vi "Width test.vi"(7 "error in":errorcluster) -> (27 "error out":errorcluster)   [LabVIEW 2014]
panel:
  in  "File Path":path=path "D:/leizhihong/胶水图片/透明胶水检测/IMG0003.bmp"
  in  "Settings":T1={"Contrast"=60, "Filter width"=5, "Steepness"=13, "Subsampling Ratio"=25, "Show Search Area"=TRUE, "Show Search Lines"=TRUE, "Show Edges Found"=TRUE, "Show Result"=TRUE}
  out "Distance":sgl
  in  "确定":bool
  in  "ROI":bool
  in  "停止":bool
  out "Image Out":T2(plugin-control)
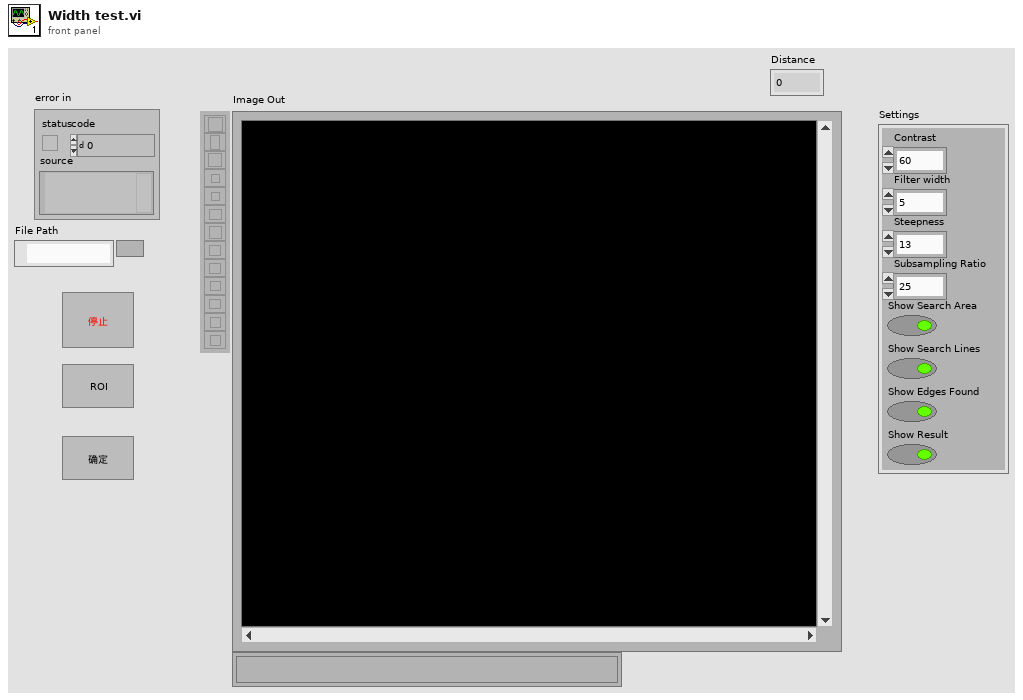
[diagram p1: front panel]
types:
  T1 = cluster{"Contrast":i32, "Filter width":i32, "Steepness":i32, "Subsampling Ratio":u32, "Show Search Area":bool, "Show Search Lines":bool, "Show Edges Found":bool, "Show Result":bool}
  T2 = typedef "IMAQ Image.ctl" = refnum<image>
  T3 = typedef "Image Type" = u32
  T4 = cluster{"Global Rectangle":i32[], "Contours":cluster{"Contour Type":u32, "ROI Type":u32, "Points":i32[]}[]}
  T5 = cluster{"Global Rectangle":i32[], "Contours":cluster{"ID":enum32{"External", "Internal"}, "Type":u32, "Coordinates":i32[]}[]}
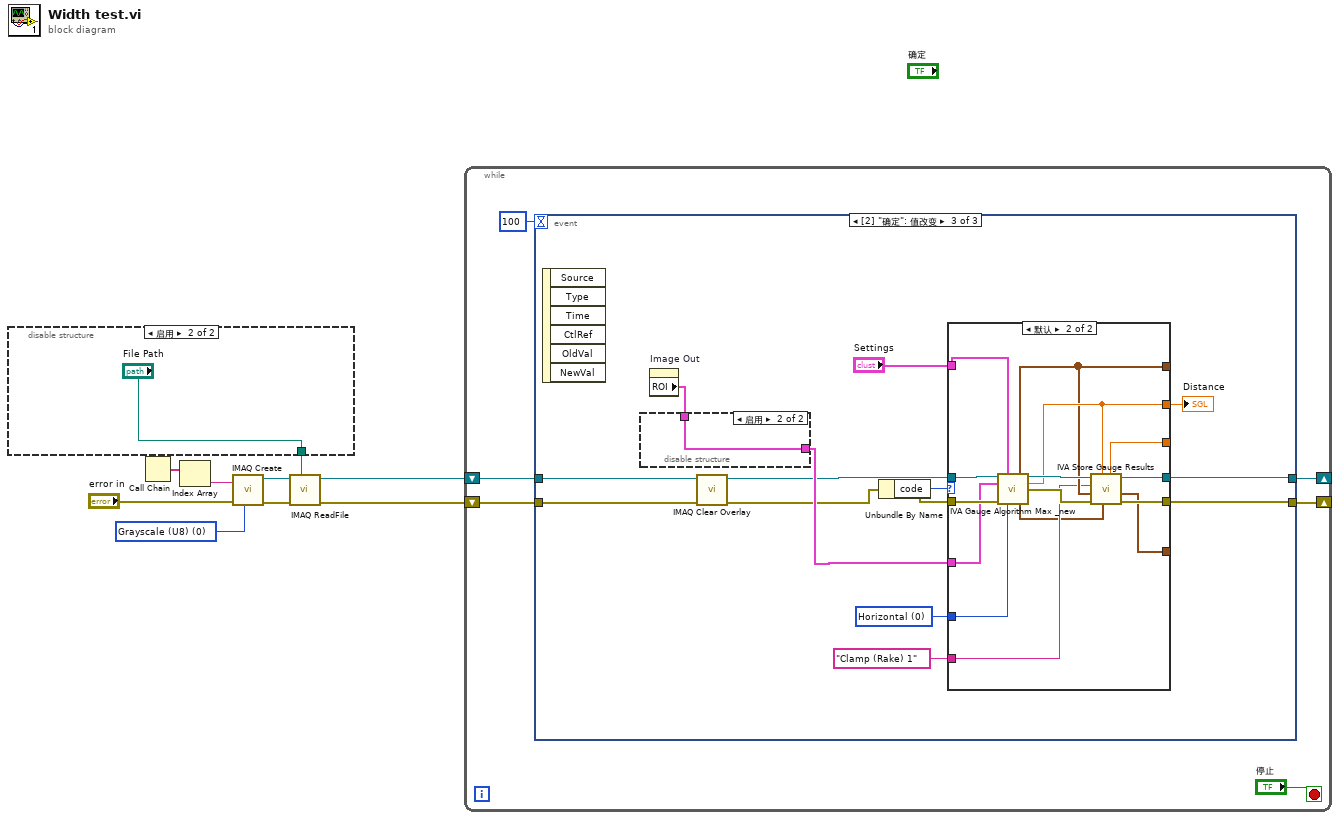
[diagram p0: block diagram]
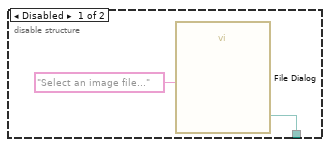
[diagram p2: hidden frame]
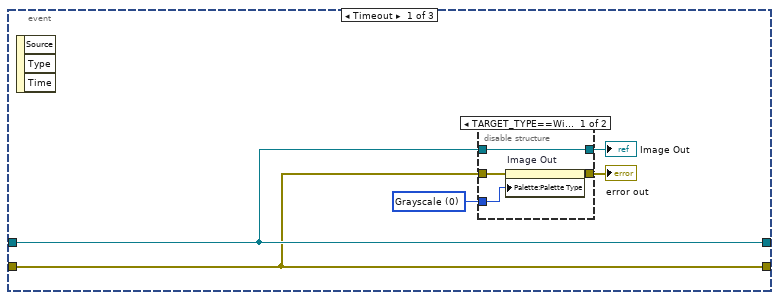
[diagram p3: hidden frame]
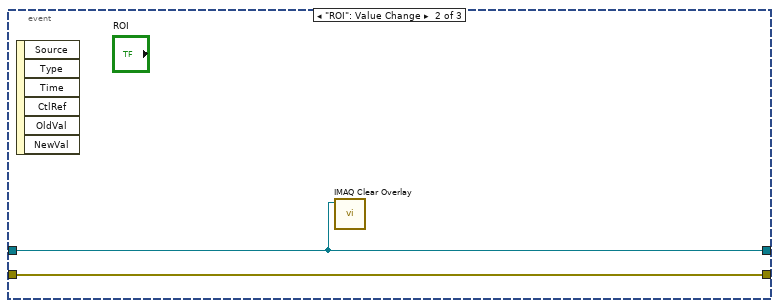
[diagram p5: hidden frame]
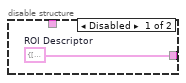
[diagram p6: hidden frame]
diagram:
  w2 = T3 0 items=["Grayscale (U8)", "Grayscale (I16)", "Grayscale (SGL)", "Complex (CSG)", "RGB (U32)", "HSL (U32)", "RGB (U64)", "Grayscale (U16)"] ("Image Type")
  n1 = disable-structure shown="启用" {
    disable-tunnel: [w10 "File Path"] -> w3
    frame Disabled {
      n2 = call "File Dialog"("prompt"="Select an image file...") -> ("selected path"=w10:path)  [unwired: 6 in, 8 out]
    }
    frame Enabled {
    }
  }
  n3 = Call Chain() -> (call chain=w5:string[])
  n4 = Index Array(array=w5) -> (element=w4:string)  [unwired: 1 in]
  n5 = call "IMAQ Create"("Image Name"=w4, "Image Type"=w2, "error in (no error)"="error in") -> ("New Image"=w8:T2, "error out"=w7:errorcluster)  [unwired: 1 in, 1 out]
  n6 = call "IMAQ ReadFile"("File Path"=w3, "error in (no error)"=w7, "Image"=w8) -> ("error out"=w9:errorcluster, "Image Out"=w1:T2)  [unwired: 2 in, 5 out]
  n7 = while {
    shift-right: [w16] -> _
    shift-left: w9 -> [w18]
    shift-right: [w15] -> _
    shift-left: w1 -> [w17]
    stop <- "停止" stop-if-true
    n8 = event shown="[2] \"确定\": 值改变" {
      selector: _ -> [_ _ _]
      dyn-events: _ -> [_ _ _]
      timeout: 100 -> [_ _ _]
      tunnel: w18 -> [w19 w31 w33]
      tunnel: w17 -> [w20 w30 w35]
      tunnel: [w19 w31 w38] -> w16
      tunnel: [w20 w30 w39] -> w15
      event Timeout {
        w23 = u32 0 items=["Grayscale", "Binary", "Gradient", "Rainbow", "Temperature", "User Defined"] ("Palette")
        n9 = event-data() -> ()  [unwired: 1 in, 3 out]
        n10 = disable-structure "条件禁用结构" shown="TARGET_TYPE==Windows" {
          disable-tunnel: w19 -> [w27 w28]
          disable-tunnel: [w26 w28] -> w21
          disable-tunnel: w20 -> [w25 w29]
          disable-tunnel: [w25 w29] -> w22
          disable-tunnel: w23 -> [w24 _]
          frame condition #0 (active) {
            n11 = property on="Image Out" class="ImageControl"(error in=w27, "Palette:Palette Type"=w24) -> (error out=w26:errorcluster)  [unwired: 1 in, 1 out]
          }
          frame condition #1 {
          }
        }
        "error out" <- w21
        "Image Out" <- w22
      }
      event "ROI": Value Change {
        n12 = event-data() -> ()  [unwired: 1 in, 6 out]
        n13 = call "IMAQ Clear Overlay"("Image"=w30) -> ()  [unwired: 9 in, 2 out]
      }
      event "确定": Value Change {
        w43 = u32 0 items=["Horizontal", "Vertical"] ("Scanning axis")
        n14 = event-data() -> ()  [unwired: 1 in, 6 out]
        n15 = property on="Image Out" class="ImageControl"() -> ("ROI"=w37:T4)  [unwired: 2 in, 2 out]
        n16 = disable-structure shown="启用" {
          disable-tunnel: [w45 w46] -> w42
          disable-tunnel: w37 -> [_ w46]
          frame Disabled {
            w45 = T5 {"Global Rectangle"=[264, 625, 475, 842], "Contours"=[{"ID"=enum."External", "Type"=12, "Coordinates"=[264, 625, 475, 842, 0]}]}  # ROI Descriptor
          }
          frame Enabled {
          }
        }
        n17 = call "IMAQ Clear Overlay"("error in (no error)"=w33, "Image"=w35) -> ("error out"=w32:errorcluster, "Image Out"=w34:T2)  [unwired: 8 in]
        n18 = Unbundle By Name(w32) -> ("code"=w41:i32)
        n19 = case "条件结构" shown="默认" w41 {
          tunnel: w34 -> [w47 w62]
          tunnel: w32 -> [_ w61]
          tunnel: "Settings" -> [_ w60]
          tunnel: w43 -> [_ w59]
          tunnel: w42 -> [_ w58]
          tunnel: [w47 w56] -> w39
          tunnel: [_ w54] -> w38
          tunnel: [_ w53] -> w36
          tunnel: [_ w52] -> _
          tunnel: [_ w51] -> _
          tunnel: [_ w50] -> _
          tunnel: "Clamp (Rake) 1" ("Step Name") -> [_ w49]
          frame -1074396199, -1074396198 {
            # "Discard Coordinate System Error"
          }
          frame Default {
            n20 = call "IVA Gauge Algorithm Max _new.vi"("Image"=w62, "Settings"=w60, "ROI Descriptor"=w58, "error in (no error)"=w61, "Scanning axis"=w59) -> ("Points of Contact"=w52:cluster{"X":sgl, "Y":sgl}[], "Image Out"=w57:T2, "Distance"=w53:sgl, "error out"=w55:errorcluster, "Distance Points"=w48:cluster{"X":sgl, "Y":sgl}[])  [unwired: 4 in, 2 out]
            n21 = call <vilib>:"IVA Store Gauge Results.vi"("Distance Points"=w48, "Distance"=w53, "error in (no error)"=w55, "Points of Contact"=w52, "Step Name"=w49, "Image in"=w57) -> ("error out"=w54:errorcluster, "Points of Contact (calibrated)"=w50:cluster{"X":sgl, "Y":sgl}[], "Image dup"=w56:T2, "Distance (calibrated)"=w51:sgl)  [unwired: 2 out]
          }
        }
        "Distance" <- w36
      }
    }
  }
